vi "PosibilProiectPS (1).vi"() -> ()   [LabVIEW 2020]
uses:
  <vilib>/Analysis/5stat.llb/RMS (DBL).vi
  <vilib>/Utility/file.llb/Read Delimited Spreadsheet (DBL).vi
  <vilib>/measure/matone.llb/Extract Multiple Tone Information 1 Chan.vi
  <vilib>/measure/matone.llb/Harmonic Distortion Analyzer 1 Chan.vi
  <vilib>/measure/NI_MAPro.lvlib
  <vilib>/Analysis/NI_AALPro.lvlib
panel:
  out "Grafic energia totala kWh 3":dbl(graph)
  out "Energia totala kWh 3":dbl
  out "Grafic energia totala Ws 3":dbl(graph)
  out "Energia totala Ws 3":dbl
  out "Grafic energia totala kWh 2":dbl(graph)
  out "Energia totala kWh 2":dbl
  out "Grafic energia totala Ws 2":dbl(graph)
  out "Energia totala Ws 2":dbl
  out "Reprezentare grafica 3":dbl[][](graph)
  out "Reprezentare grafica 2":dbl[][](graph)
  out "Reprezentare grafica":dbl[][](graph)
  out "Grafic energia totala kWh":dbl(graph)
  out "Energia totala kWh":dbl
  out "Grafic energia totala Ws":dbl(graph)
  out "Energia totala Ws":dbl
  out "Timp[h]  3":dbl format="%.15f"
  in  "Calculul energiei":string
  in  "Calculul puteriilor":string
  out "Grafic energia reactiva Q [kVAh] 2":dbl(graph)
  out "Eq[kVAh]  6":dbl
  out "Q [kVA] 4":dbl
  out "P [kW] 4":dbl
  out "Grafic energia activa  P[kWh]":dbl(graph)
  out "Ep[kWh] 7":dbl
  out "Grafic energia aparenta S[kVAh]  4":dbl(graph)
  out "Es[kVAh] 7":dbl
  out "S [kVA] 4":dbl
  out "Grafic energia deformata  D[kVADh] 4":dbl(graph)
  out "Ed[kVADh] 7":dbl
  out "D [kVAD] 4":dbl
  in  "Calulul energiei":string
  in  "Calculul puteriilor":string
  out "Timp[h]  2":dbl format="%.15f"
  out "S [kVA] 4":dbl
  out "Q [kVA] 4":dbl
  out "Grafic energia reactiva Q[kVAh] 3":dbl(graph)
  out "Eq[kVAh]  4":dbl
  out "P [kW] 4":dbl
  out "Grafic energia activa  P[kWh] 4":dbl(graph)
  out "Ep[kWh] 5":dbl
  out "Grafic energia aparenta S[kVAh]  3":dbl(graph)
  out "Es[kVAh] 5":dbl
  out "Grafic energia deformata  D[kVADh]":dbl(graph)
  out "Ed[kVADh]":dbl
  out "D [kVAD]":dbl
  in  "Calculul energiei":string
  in  "Calculul puterilor":u16(ring)
  out "Q [kVA]":dbl
  out "Grafic energia reactiva Q[kVAh]":dbl(graph)
  out "Eq[kVAh]":dbl
  out "Grafic energia aparenta S[kVAh]":dbl(graph)
  out "Es[kVAh]":dbl
  out "S [kVA]":dbl
  out "Grafic energia activa  P [kWh]":dbl(graph)
  out "Ep[kWh]":dbl
  out "P [kW]":dbl
  out "Timp[h]":dbl format="%.15f"
  out "Grafic energia deformata  D[kVADh]":dbl(graph)
  out "D [kVAD]":dbl
  out "Ed[kVADh]":dbl
  in  "Fisierul 3\nSistem de iluminat":path
  in  "Fisierul 2\nMotor electric alimentat prin convertor de frecventa":path
  in  "Fisierul 1\nMotor electric alimentat direct la retea":path
  out "Timp [s] 3":i32
  out "Grafic energia deformata  D[VADs] 3":dbl(graph)
  out "Grafic energia aparenta S[VAs]  3":dbl(graph)
  out "Grafic energia reactiva Q [VAs]":dbl(graph)
  out "Grafic energia activa  P[Ws] 3":dbl(graph)
  out "3rd harmonic graph 3":waveform(dbl)(graph)
  in  "Calculul puteriilor":string
  in  "Calculul energiei":string
  out "Ed[VADs] 6":dbl
  out "Eq[VAs]  5":dbl
  out "Ep[Ws] 6":dbl
  out "Es[VAs] 6":dbl
  out "Q [VA] 3":dbl
  out "D [VAD] 3":dbl
  out "P [W] 3":dbl
  out "S [VA] 3":dbl
  out "rms curent fundamental 3":dbl format="%0.2f"
  out "rms value voltage 3":dbl format="%0.2f"
  out "rms current 3rd harmonic 3":dbl format="%0.2f"
  out "?":waveform(dbl)
  out "fundamental graph 3":waveform(dbl)(graph)
  out "3rd current harmonic signal  3":waveform(dbl)
  out "multiple tone information 3":T1(array[cluster]) {"detected phase (deg)" format="%_6g"; "detected amplitude" format="%_6p"; "detected frequency" format="%_6p"}
  in  "export mode 6":T2(ring)=enum."harmonics only"
  in  "export mode 5":T2(ring)=enum."fundamental signal"
  out "input signal graph 3":dbl[](graph)
  in  "Nr_spire 3":dbl=5.0
  out "Tabel complet 3":dbl[][](array[numeric])
  out "Timp [s]2":i32
  out "Grafic energia deformata  D[VADs ]":dbl(graph)
  out "Grafic energia aparenta S[VAs]  2":dbl(graph)
  out "Grafic energia reactiva Q[VAs] 2":dbl(graph)
  out "Grafic energia activa  P[Ws] 2":dbl(graph)
  out "3rd harmonic graph 2":waveform(dbl)(graph)
  in  "Calculul puteriilor":string
  in  "Calulul energiei":string
  out "Ed[VADs] 4":dbl
  out "Eq[VAs]  3":dbl
  out "Ep[Ws] 4":dbl
  out "Es[VAs] 4":dbl
  out "Q [VA] 2":dbl
  out "D [VAD] 2":dbl
  out "P [W] 2":dbl
  out "S [VA] 2":dbl
  out "rms curent fundamental 2":dbl format="%0.2f"
  out "rms value voltage 2":dbl format="%0.2f"
  out "rms current 3rd harmonic 2":dbl format="%0.2f"
  out "?":waveform(dbl)
  out "fundamental graph 2":waveform(dbl)(graph)
  out "3rd current harmonic signal  2":waveform(dbl)
  out "multiple tone information 2":T1(array[cluster]) {"detected phase (deg)" format="%_6g"; "detected amplitude" format="%_6p"; "detected frequency" format="%_6p"}
  in  "export mode 4":T2(ring)=enum."harmonics only"
  in  "export mode 3":T2(ring)=enum."fundamental signal"
  out "input signal graph 2":dbl[](graph)
  in  "Nr_spire 2":dbl=5.0
  out "Tabel complet 2":dbl[][](array[numeric])
  out "Timp[s]":i32
  in  "stop":bool
  out "Grafic energia deformata  D[VADs]":dbl(graph)
  out "Grafic energia aparenta S[VAs]":dbl(graph)
  out "Grafic energia reactiva  Q[VAs]":dbl(graph)
  out "Grafic energia activa  P[Ws]":dbl(graph)
  out "3rd harmonic graph":waveform(dbl)(graph)
  in  "Calculul puterilor":string
  in  "Calculul energiei":string
  out "Ed[VADs] 2":dbl
  out "Eq[VAs]  2":dbl
  out "Ep[Ws] 2":dbl
  out "Es[VAs] 2":dbl
  out "Q [VA]":dbl
  out "D [VAD]":dbl
  out "P [W]":dbl
  out "S [VA]":dbl
  out "rms curent fundamental":dbl format="%0.2f"
  out "rms value voltage":dbl format="%0.2f"
  out "rms current 3rd harmonic":dbl format="%0.2f"
  out "?":waveform(dbl)
  out "fundamental graph":waveform(dbl)(graph)
  out "3rd current harmonic signal":waveform(dbl)
  out "multiple tone information":T1(array[cluster]) {"detected phase (deg)" format="%_6g"; "detected amplitude" format="%_6p"; "detected frequency" format="%_6p"}
  in  "export mode 2":T2(ring)=enum."harmonics only"
  in  "export mode":T2(ring)=enum."fundamental signal"
  out "input signal graph":dbl[](graph)
  in  "Nr_spire":dbl=5.0
  out "Tabel complet":dbl[][](array[numeric])
  # "Graficele energiei in functie de timpul in secunde"
  # "Graficele energiei in functie de timpul in ore"
  # "Graficele energiei totale in Wsecunde /kW ore"
  # "Graficele energiei in functie de timpul in secunde"
  # "Graficele energiei in functie de timpul in ore"
  # "Graficele energiei totale in Wsecunde /kW ore"
  # "Graficele energiei in functie de timpul in secunde"
  # "Graficele energiei in functie de timpul in ore"
  # "Graficele energiei totale in Wsecunde /kW ore"
types:
  T1 = cluster{"detected frequency":dbl, "detected amplitude":dbl, "detected phase (deg)":dbl}[]
  T2 = enum16{"none", "input signal", "fundamental signal", "residual signal", "harmonics only", "noise and spurs"}
  T3 = cluster{"exported time signal":waveform(dbl), "exported spectrum (dB)":cluster{"f0":dbl, "df":dbl, "dB Spectrum (Hann)":dbl[]}}
  T4 = cluster{"detected frequency":dbl, "detected amplitude":dbl, "detected phase (deg)":dbl}
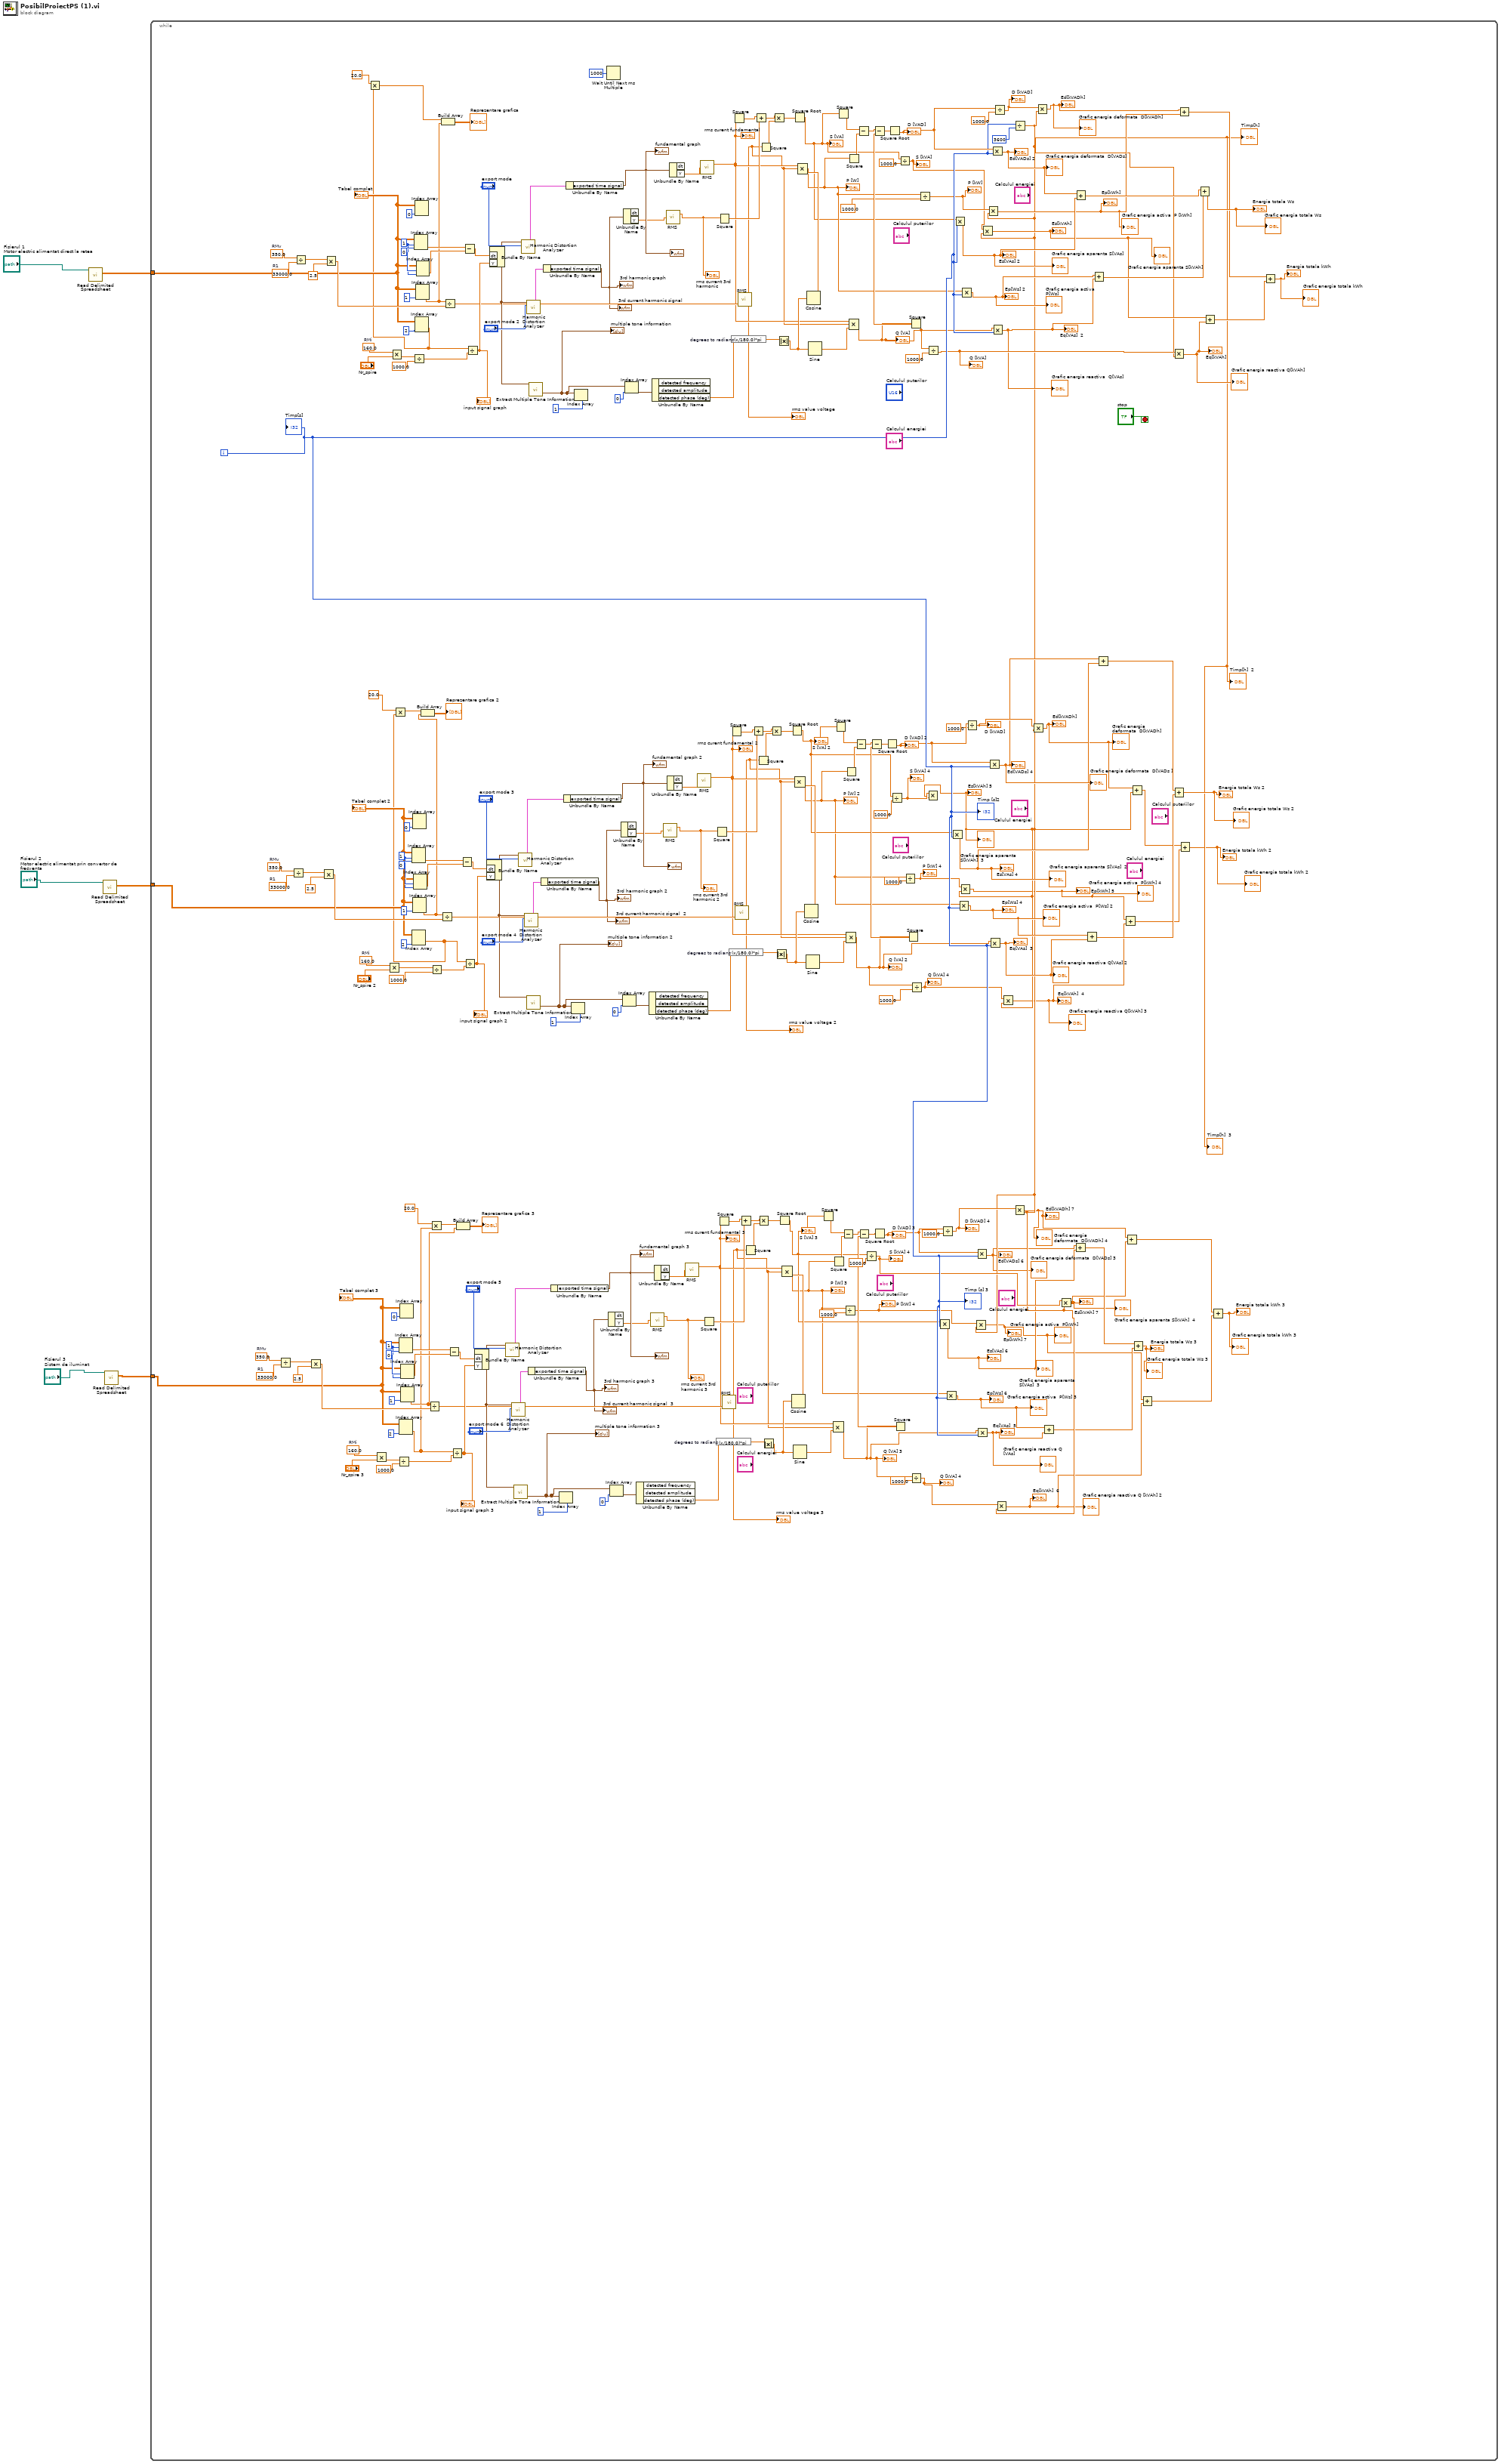
[diagram p0: block diagram]
diagram:
  n1 = call-poly <vilib>:"Read Delimited Spreadsheet.vi"("file path (dialog if empty)"="Fisierul 1\nMotor electric alimentat direct la retea") -> ("all rows"=w6:dbl[][])  [unwired: 9 in, 5 out]
  n2 = call-poly <vilib>:"Read Delimited Spreadsheet.vi"("file path (dialog if empty)"="Fisierul 2\nMotor electric alimentat prin convertor de frecventa") -> ("all rows"=w5:dbl[][])  [unwired: 9 in, 5 out]
  n3 = call-poly <vilib>:"Read Delimited Spreadsheet.vi"("file path (dialog if empty)"="Fisierul 3\nSistem de iluminat") -> ("all rows"=w4:dbl[][])  [unwired: 9 in, 5 out]
  n4 = while {
    tunnel: w6 -> [w211]
    tunnel: w5 -> [w154]
    tunnel: w4 -> [w102]
    i -> [w99]
    stop <- "stop" stop-if-true
    w143 = 160.0  # RMi
    w148 = 0 ("index (row)")
    w147 = 1 ("index (row)")
    w152 = 350.0  # RMv
    w153 = 33000.0  # R1
    w195 = 160.0  # RMi
    w200 = 0 ("index (row)")
    w199 = 1 ("index (row)")
    w204 = 350.0  # RMv
    w205 = 33000.0  # R1
    w249 = 160.0  # RMi
    w254 = 0 ("index (row)")
    w253 = 1 ("index (row)")
    w258 = 350.0  # RMv
    w259 = 33000.0  # R1
    n5 = Divide(x=w152, y=w153) -> (x/y=w151:dbl)
    n6 = Divide(x=w204, y=w205) -> (x/y=w203:dbl)
    n7 = Divide(x=w258, y=w259) -> (x/y=w257:dbl)
    n8 = Multiply(x=w151, y=2.5) -> (x*y=w145:dbl)
    n9 = Multiply(x=w203, y=2.5) -> (x*y=w197:dbl)
    n10 = Multiply(x=w257, y=2.5) -> (x*y=w251:dbl)
    n11 = Multiply(x=w143, y="Nr_spire 3") -> (x*y=w140:dbl)
    n12 = Multiply(x=w195, y="Nr_spire 2") -> (x*y=w192:dbl)
    n13 = Multiply(x=w249, y="Nr_spire") -> (x*y=w246:dbl)
    n14 = Divide(x=w140, y=1000.0) -> (x/y=w139:dbl)
    n15 = Index Array(array=w102, index (row)=w147, index (col)=w148) -> (element=w105:dbl)
    n16 = Index Array(array=w102, index (col)=2 ("disabled index (col)")) -> (element=w35:dbl[])  [unwired: 1 in]
    n17 = Index Array(array=w102, index (row)=0) -> ()  [unwired: 1 in, 1 out]
    n18 = Index Array(array=w102, index (col)=1 ("disabled index (col)")) -> (element=w36:dbl[])  [unwired: 1 in]
    n19 = Index Array(array=w102, index (row)=w148, index (col)=w147) -> (element=w149:dbl)
    n20 = Index Array(array=w154, index (row)=w199, index (col)=w200) -> (element=w157:dbl)
    n21 = Index Array(array=w154, index (col)=2 ("disabled index (col)")) -> (element=w40:dbl[])  [unwired: 1 in]
    n22 = Multiply(x=20.0 ("y"), y=w40) -> (x*y=w43:dbl[])
    n23 = Divide(x=w246, y=1000.0) -> (x/y=w245:dbl)
    n24 = Index Array(array=w154, index (row)=0) -> ()  [unwired: 1 in, 1 out]
    n25 = Index Array(array=w154, index (col)=1 ("disabled index (col)")) -> (element=w41:dbl[])  [unwired: 1 in]
    n26 = Index Array(array=w154, index (row)=w200, index (col)=w199) -> (element=w201:dbl)
    n27 = Index Array(array=w211, index (row)=w253, index (col)=w254) -> (element=w210:dbl)
    n28 = Index Array(array=w211, index (col)=2 ("disabled index (col)")) -> (element=w46:dbl[])  [unwired: 1 in]
    n29 = Multiply(x=20.0 ("y"), y=w46) -> (x*y=w47:dbl[])
    n30 = Index Array(array=w211, index (row)=0) -> ()  [unwired: 1 in, 1 out]
    n31 = Index Array(array=w211, index (col)=1 ("disabled index (col)")) -> (element=w45:dbl[])  [unwired: 1 in]
    n32 = Index Array(array=w211, index (row)=w254, index (col)=w253) -> (element=w255:dbl)
    n33 = Build Array(w43, w41) -> (→"Reprezentare grafica 2":dbl[][])
    n34 = Divide(x=w36, y=w145) -> (x/y=w123:dbl[])
    n35 = Multiply(x=20.0 ("y"), y=w35) -> (x*y=w38:dbl[])
    n36 = Divide(x=w192, y=1000.0) -> (x/y=w191:dbl)
    n37 = Divide(x=w41, y=w197) -> (x/y=w175:dbl[])
    n38 = Build Array(w47, w45) -> (→"Reprezentare grafica":dbl[][])
    n39 = Divide(x=w45, y=w251) -> (x/y=w229:dbl[])
    n40 = Subtract(x=w105, y=w149) -> (x-y=w104:dbl)
    n41 = Divide(x=w35, y=w139) -> (x/y=w138:dbl[])
    "input signal graph 3" <- w138
    n42 = Build Array(w38, w36) -> (→"Reprezentare grafica 3":dbl[][])
    n43 = Subtract(x=w157, y=w201) -> (x-y=w156:dbl)
    n44 = Subtract(x=w210, y=w255) -> (x-y=w209:dbl)
    n45 = Divide(x=w40, y=w191) -> (x/y=w190:dbl[])
    "input signal graph 2" <- w190
    n46 = Divide(x=w46, y=w245) -> (x/y=w244:dbl[])
    "input signal graph" <- w244
    n47 = Bundle By Name("dt"=w104, "Y"=w138) -> (w135:waveform(dbl))  [unwired: 1 in]
    n48 = Bundle By Name("dt"=w156, "Y"=w190) -> (w187:waveform(dbl))  [unwired: 1 in]
    n49 = Bundle By Name("dt"=w209, "Y"=w244) -> (w241:waveform(dbl))  [unwired: 1 in]
    n50 = call-poly <vilib>:"Harmonic Distortion Analyzer.vi"("export mode"="export mode 5", "signal in"=w135) -> ("exported signals"=w134:T3)  [unwired: 4 in, 5 out]
    n51 = call-poly <vilib>:"Harmonic Distortion Analyzer.vi"("export mode"="export mode 6", "signal in"=w135) -> ("exported signals"=w133:T3)  [unwired: 4 in, 5 out]
    n52 = call-poly <vilib>:"Extract Multiple Tone Information.vi"("time signal in"=w135) -> ("multiple tone information"=w131:T1)  [unwired: 12 in, 2 out]
    "multiple tone information 3" <- w131
    n53 = call-poly <vilib>:"Harmonic Distortion Analyzer.vi"("export mode"="export mode 3", "signal in"=w187) -> ("exported signals"=w186:T3)  [unwired: 4 in, 5 out]
    n54 = call-poly <vilib>:"Harmonic Distortion Analyzer.vi"("export mode"="export mode", "signal in"=w241) -> ("exported signals"=w240:T3)  [unwired: 4 in, 5 out]
    n55 = call-poly <vilib>:"Harmonic Distortion Analyzer.vi"("export mode"="export mode 4", "signal in"=w187) -> ("exported signals"=w185:T3)  [unwired: 4 in, 5 out]
    n56 = call-poly <vilib>:"Extract Multiple Tone Information.vi"("time signal in"=w187) -> ("multiple tone information"=w183:T1)  [unwired: 12 in, 2 out]
    "multiple tone information 2" <- w183
    n57 = call-poly <vilib>:"Harmonic Distortion Analyzer.vi"("export mode"="export mode 2", "signal in"=w241) -> ("exported signals"=w239:T3)  [unwired: 4 in, 5 out]
    n58 = Unbundle By Name(w133) -> ("exported time signal"=w103:waveform(dbl))
    "3rd current harmonic signal  3" <- w103
    "3rd harmonic graph 3" <- w103
    n59 = call-poly <vilib>:"Extract Multiple Tone Information.vi"("time signal in"=w241) -> ("multiple tone information"=w237:T1)  [unwired: 12 in, 2 out]
    "multiple tone information" <- w237
    n60 = Unbundle By Name(w185) -> ("exported time signal"=w155:waveform(dbl))
    "3rd current harmonic signal  2" <- w155
    "3rd harmonic graph 2" <- w155
    n61 = Unbundle By Name(w239) -> ("exported time signal"=w208:waveform(dbl))
    "3rd current harmonic signal" <- w208
    "3rd harmonic graph" <- w208
    n62 = Unbundle By Name(w134) -> ("exported time signal"=w128:waveform(dbl))
    "fundamental graph 3" <- w128
    "?" <- w128
    n63 = Index Array(array=w131, index=1) -> ()  [unwired: 1 out]
    n64 = Unbundle By Name(w186) -> ("exported time signal"=w180:waveform(dbl))
    "fundamental graph 2" <- w180
    "?" <- w180
    n65 = Unbundle By Name(w240) -> ("exported time signal"=w234:waveform(dbl))
    "fundamental graph" <- w234
    "?" <- w234
    n66 = Index Array(array=w183, index=1) -> ()  [unwired: 1 out]
    n67 = Index Array(array=w237, index=1) -> ()  [unwired: 1 out]
    n68 = Wait Until Next ms Multiple(millisecond multiple=u32 1000) -> ()  [unwired: 1 out]
    n69 = Unbundle By Name(w103) -> ("Y"=w127:dbl[])  [unwired: 1 out]
    n70 = Index Array(array=w131, index=0) -> (element=w129:T4)
    n71 = Unbundle By Name(w155) -> ("Y"=w179:dbl[])  [unwired: 1 out]
    n72 = Index Array(array=w183, index=0) -> (element=w181:T4)
    n73 = Unbundle By Name(w208) -> ("Y"=w233:dbl[])  [unwired: 1 out]
    n74 = Index Array(array=w237, index=0) -> (element=w235:T4)
    n75 = Unbundle By Name(w129) -> ("detected phase (deg)"=w124:dbl)  [unwired: 2 out]
    n76 = Unbundle By Name(w181) -> ("detected phase (deg)"=w176:dbl)  [unwired: 2 out]
    n77 = call-poly <vilib>:"RMS.vi"("X"=w127) -> ("rms value"=w125:dbl)  [unwired: 1 out]
    "rms current 3rd harmonic 3" <- w125
    n78 = Unbundle By Name(w235) -> ("detected phase (deg)"=w230:dbl)  [unwired: 2 out]
    n79 = Unbundle By Name(w128) -> ("Y"=w126:dbl[])  [unwired: 1 out]
    n80 = call-poly <vilib>:"RMS.vi"("X"=w179) -> ("rms value"=w177:dbl)  [unwired: 1 out]
    "rms current 3rd harmonic 2" <- w177
    n81 = call-poly <vilib>:"RMS.vi"("X"=w233) -> ("rms value"=w231:dbl)  [unwired: 1 out]
    "rms current 3rd harmonic" <- w231
    n82 = Unbundle By Name(w180) -> ("Y"=w178:dbl[])  [unwired: 1 out]
    n83 = Unbundle By Name(w234) -> ("Y"=w232:dbl[])  [unwired: 1 out]
    n84 = call-poly <vilib>:"RMS.vi"("X"=w126) -> ("rms value"=w110:dbl)  [unwired: 1 out]
    "rms curent fundamental 3" <- w110
    n85 = call-poly <vilib>:"RMS.vi"("X"=w178) -> ("rms value"=w162:dbl)  [unwired: 1 out]
    "rms curent fundamental 2" <- w162
    n86 = call-poly <vilib>:"RMS.vi"("X"=w232) -> ("rms value"=w216:dbl)  [unwired: 1 out]
    "rms curent fundamental" <- w216
    n87 = Square(x=w125) -> (x^2=w119:dbl)
    n88 = Square(x=w177) -> (x^2=w171:dbl)
    n89 = expression code="(x/180.0)*pi" "degrees to radians"(w124) -> (w122:dbl)
    n90 = Square(x=w110) -> (x^2=w120:dbl)
    n91 = Square(x=w231) -> (x^2=w225:dbl)
    n92 = call-poly <vilib>:"RMS.vi"("X"=w123) -> ("rms value"=w109:dbl)  [unwired: 1 out]
    "rms value voltage 3" <- w109
    n93 = expression code="(x/180.0)*pi" "degrees to radians"(w176) -> (w174:dbl)
    n94 = Square(x=w162) -> (x^2=w172:dbl)
    n95 = expression code="(x/180.0)*pi" "degrees to radians"(w230) -> (w228:dbl)
    n96 = Square(x=w216) -> (x^2=w226:dbl)
    n97 = call-poly <vilib>:"RMS.vi"("X"=w175) -> ("rms value"=w161:dbl)  [unwired: 1 out]
    "rms value voltage 2" <- w161
    n98 = call-poly <vilib>:"RMS.vi"("X"=w229) -> ("rms value"=w215:dbl)  [unwired: 1 out]
    "rms value voltage" <- w215
    n99 = Add(x=w120, y=w119) -> (x+y=w118:dbl)
    n100 = Square(x=w109) -> (x^2=w117:dbl)
    n101 = Add(x=w172, y=w171) -> (x+y=w170:dbl)
    n102 = Add(x=w226, y=w225) -> (x+y=w224:dbl)
    n103 = Square(x=w161) -> (x^2=w169:dbl)
    n104 = Multiply(x=w118, y=w117) -> (x*y=w116:dbl)
    n105 = Square(x=w215) -> (x^2=w223:dbl)
    n106 = Absolute Value(x=w122) -> (abs(x)=w121:dbl)
    n107 = Multiply(x=w170, y=w169) -> (x*y=w168:dbl)
    n108 = Multiply(x=w224, y=w223) -> (x*y=w222:dbl)
    n109 = Absolute Value(x=w174) -> (abs(x)=w173:dbl)
    n110 = Absolute Value(x=w228) -> (abs(x)=w227:dbl)
    n111 = Square Root(x=w116) -> (sqrt(x)=w72:dbl)
    "S [VA] 3" <- w72
    n112 = Square Root(x=w168) -> (sqrt(x)=w84:dbl)
    "S [VA] 2" <- w84
    n113 = Cosine(x=w121) -> (cos(x)=w115:dbl)
    n114 = Compound Arithmetic op=MULTIPLY(w110, w109, w115) -> (w69:dbl)
    "P [W] 3" <- w69
    n115 = Square Root(x=w222) -> (sqrt(x)=w93:dbl)
    "S [VA]" <- w93
    n116 = Sine(x=w121) -> (sin(x)=w108:dbl)
    n117 = Cosine(x=w173) -> (cos(x)=w167:dbl)
    n118 = Compound Arithmetic op=MULTIPLY(w162, w161, w167) -> (w83:dbl)
    "P [W] 2" <- w83
    n119 = Sine(x=w173) -> (sin(x)=w160:dbl)
    n120 = Cosine(x=w227) -> (cos(x)=w221:dbl)
    n121 = Compound Arithmetic op=MULTIPLY(w216, w215, w221) -> (w96:dbl)
    "P [W]" <- w96
    n122 = Sine(x=w227) -> (sin(x)=w214:dbl)
    n123 = Square(x=w72) -> (x^2=w114:dbl)
    n124 = Square(x=w69) -> (x^2=w113:dbl)
    n125 = Compound Arithmetic op=MULTIPLY(w110, w109, w108) -> (w66:dbl)
    "Q [VA] 3" <- w66
    n126 = Square(x=w84) -> (x^2=w166:dbl)
    n127 = Square(x=w93) -> (x^2=w220:dbl)
    n128 = Subtract(x=w114, y=w113) -> (x-y=w112:dbl)
    n129 = Divide(x=w69, y=1000.0 ("x")) -> (x/y=w67:dbl)
    "P [kW] 4" <- w67
    n130 = Square(x=w83) -> (x^2=w165:dbl)
    n131 = Compound Arithmetic op=MULTIPLY(w162, w161, w160) -> (w80:dbl)
    "Q [VA] 2" <- w80
    n132 = Square(x=w96) -> (x^2=w219:dbl)
    n133 = Compound Arithmetic op=MULTIPLY(w216, w215, w214) -> (w90:dbl)
    "Q [VA]" <- w90
    n134 = Subtract(x=w166, y=w165) -> (x-y=w164:dbl)
    n135 = Subtract(x=w220, y=w219) -> (x-y=w218:dbl)
    n136 = Divide(x=w72, y=1000.0 ("x")) -> (x/y=w70:dbl)
    "S [kVA] 4" <- w70
    n137 = Divide(x=w84, y=1000.0 ("x/y")) -> (x/y=w76:dbl)
    "S [kVA] 4" <- w76
    n138 = Square(x=w66) -> (x^2=w107:dbl)
    n139 = Subtract(x=w112, y=w107) -> (x-y=w111:dbl)
    n140 = Square Root(x=w111) -> (sqrt(x)=w75:dbl)
    "D [VAD] 3" <- w75
    n141 = Divide(x=w93, y=1000.0) -> (x/y=w91:dbl)
    "S [kVA]" <- w91
    n142 = Divide(x=w83, y=1000.0) -> (x/y=w81:dbl)
    "P [kW] 4" <- w81
    n143 = Square(x=w80) -> (x^2=w159:dbl)
    n144 = Subtract(x=w164, y=w159) -> (x-y=w163:dbl)
    n145 = Square Root(x=w163) -> (sqrt(x)=w87:dbl)
    "D [VAD] 2" <- w87
    n146 = Square(x=w90) -> (x^2=w213:dbl)
    n147 = Subtract(x=w218, y=w213) -> (x-y=w217:dbl)
    n148 = Square Root(x=w217) -> (sqrt(x)=w101:dbl)
    "D [VAD]" <- w101
    n149 = Divide(x=w66, y=1000.0) -> (x/y=w64:dbl)
    "Q [kVA] 4" <- w64
    n150 = Divide(x=w80, y=1000.0) -> (x/y=w78:dbl)
    "Q [kVA] 4" <- w78
    n151 = Divide(x=w96, y=1000.0) -> (x/y=w94:dbl)
    "P [kW]" <- w94
    n152 = Divide(x=w90, y=1000.0) -> (x/y=w88:dbl)
    "Q [kVA]" <- w88
    n153 = Multiply(x=w72, y=w99) -> (x*y=w19:dbl)
    "Es[VAs] 6" <- w19
    "Grafic energia aparenta S[VAs]  3" <- w19
    n154 = Divide(x=w75, y=1000.0) -> (x/y=w73:dbl)
    "D [kVAD] 4" <- w73
    n155 = Multiply(x=w69, y=w99) -> (x*y=w18:dbl)
    "Ep[Ws] 6" <- w18
    "Grafic energia activa  P[Ws] 3" <- w18
    n156 = Multiply(x=w84, y=w99) -> (x*y=w33:dbl)
    "Es[VAs] 4" <- w33
    "Grafic energia aparenta S[VAs]  2" <- w33
    n157 = Multiply(x=w93, y=w99) -> (x*y=w62:dbl)
    "Es[VAs] 2" <- w62
    "Grafic energia aparenta S[VAs]" <- w62
    n158 = Multiply(x=w83, y=w99) -> (x*y=w32:dbl)
    "Ep[Ws] 4" <- w32
    "Grafic energia activa  P[Ws] 2" <- w32
    n159 = Multiply(x=w96, y=w99) -> (x*y=w61:dbl)
    "Ep[Ws] 2" <- w61
    "Grafic energia activa  P[Ws]" <- w61
    n160 = Divide(x=w87, y=1000.0) -> (x/y=w85:dbl)
    "D [kVAD]" <- w85
    n161 = Multiply(x=w75, y=w99) -> (x*y=w20:dbl)
    "Ed[VADs] 6" <- w20
    "Grafic energia deformata  D[VADs] 3" <- w20
    n162 = Multiply(x=w66, y=w99) -> (x*y=w17:dbl)
    "Eq[VAs]  5" <- w17
    "Grafic energia reactiva Q [VAs]" <- w17
    n163 = Multiply(x=w87, y=w99) -> (x*y=w34:dbl)
    "Ed[VADs] 4" <- w34
    "Grafic energia deformata  D[VADs ]" <- w34
    n164 = Multiply(x=w80, y=w99) -> (x*y=w31:dbl)
    "Eq[VAs]  3" <- w31
    "Grafic energia reactiva Q[VAs] 2" <- w31
    n165 = Multiply(x=w101, y=w99) -> (x*y=w63:dbl)
    "Ed[VADs] 2" <- w63
    "Grafic energia deformata  D[VADs]" <- w63
    n166 = Multiply(x=w90, y=w99) -> (x*y=w60:dbl)
    "Eq[VAs]  2" <- w60
    "Grafic energia reactiva  Q[VAs]" <- w60
    n167 = Divide(x=w101, y=1000.0) -> (x/y=w97:dbl)
    "D [kVAD]" <- w97
    n168 = Divide(x=w99, y=3600) -> (x/y=w26:dbl)
    "Timp[h]" <- w26
    "Es[kVAh] 5" <- w26
    "Grafic energia aparenta S[kVAh]  3" <- w26
    "Timp[h]  2" <- w26
    "Timp[h]  3" <- w26
    n169 = Multiply(x=w76, y=w26) -> ()  [unwired: 1 out]
    n170 = Multiply(x=w81, y=w26) -> (x*y=w25:dbl)
    "Ep[kWh] 5" <- w25
    "Grafic energia activa  P[kWh] 4" <- w25
    n171 = Multiply(x=w67, y=w26) -> (x*y=w11:dbl)
    "Ep[kWh] 7" <- w11
    "Grafic energia activa  P[kWh]" <- w11
    n172 = Multiply(x=w91, y=w26) -> (x*y=w53:dbl)
    "Es[kVAh]" <- w53
    "Grafic energia aparenta S[kVAh]" <- w53
    n173 = Multiply(x=w94, y=w26) -> (x*y=w55:dbl)
    "Ep[kWh]" <- w55
    "Grafic energia activa  P [kWh]" <- w55
    n174 = Multiply(x=w64, y=w26) -> (x*y=w10:dbl)
    "Eq[kVAh]  6" <- w10
    "Grafic energia reactiva Q [kVAh] 2" <- w10
    n175 = Multiply(x=w78, y=w26) -> (x*y=w24:dbl)
    "Eq[kVAh]  4" <- w24
    "Grafic energia reactiva Q[kVAh] 3" <- w24
    n176 = Multiply(x=w73, y=w26) -> (x*y=w13:dbl)
    "Ed[kVADh] 7" <- w13
    "Grafic energia deformata  D[kVADh] 4" <- w13
    n177 = Multiply(x=w85, y=w26) -> (x*y=w27:dbl)
    "Ed[kVADh]" <- w27
    "Grafic energia deformata  D[kVADh]" <- w27
    n178 = Multiply(x=w97, y=w26) -> (x*y=w56:dbl)
    "Ed[kVADh]" <- w56
    "Grafic energia deformata  D[kVADh]" <- w56
    n179 = Add(x=w18, y=w17) -> (x+y=w15:dbl)
    n180 = Multiply(x=w70, y=w26) -> (x*y=w12:dbl)
    "Es[kVAh] 7" <- w12
    "Grafic energia aparenta S[kVAh]  4" <- w12
    n181 = Add(x=w20, y=w19) -> (x+y=w16:dbl)
    n182 = Add(x=w63, y=w62) -> (x+y=w59:dbl)
    n183 = Add(x=w32, y=w31) -> (x+y=w29:dbl)
    n184 = Add(x=w61, y=w60) -> (x+y=w58:dbl)
    n185 = Add(x=w34, y=w33) -> (x+y=w30:dbl)
    n186 = Add(x=w25, y=w24) -> (x+y=w22:dbl)
    n187 = Add(x=w13, y=w12) -> (x+y=w9:dbl)
    n188 = Add(x=w27, y=w26) -> (x+y=w23:dbl)
    n189 = Add(x=w16, y=w15) -> (x+y=→"Energia totala Ws 3" →"Grafic energia totala Ws 3":dbl)
    n190 = Add(x=w11, y=w10) -> (x+y=w8:dbl)
    n191 = Multiply(x=w88, y=w26) -> (x*y=w54:dbl)
    "Eq[kVAh]" <- w54
    "Grafic energia reactiva Q[kVAh]" <- w54
    n192 = Add(x=w30, y=w29) -> (x+y=→"Energia totala Ws 2" →"Grafic energia totala Ws 2":dbl)
    n193 = Add(x=w56, y=w55) -> (x+y=w51:dbl)
    n194 = Add(x=w23, y=w22) -> (x+y=→"Energia totala kWh 2" →"Grafic energia totala kWh 2":dbl)
    n195 = Add(x=w59, y=w58) -> (x+y=→"Energia totala Ws" →"Grafic energia totala Ws":dbl)
    n196 = Add(x=w53, y=w54) -> (x+y=w52:dbl)
    n197 = Add(x=w9, y=w8) -> (x+y=→"Energia totala kWh 3" →"Grafic energia totala kWh 3":dbl)
    n198 = Add(x=w51, y=w52) -> (x+y=→"Energia totala kWh" →"Grafic energia totala kWh":dbl)
    "Tabel complet" <- w211
    "Timp[s]" <- w99
    "Tabel complet 2" <- w154
    "Timp [s]2" <- w99
    "Tabel complet 3" <- w102
    "Timp [s] 3" <- w99
  }
